vi "PrefValToXMLArray.vi"(8 "error in (no error)":errorcluster, 11 "Preferences in":refnum<class "SetListPrefs.lvclass">) -> (0 "error out":errorcluster, 2 "PrefXML":string[](array[string]), 3 "Preferences out":refnum<class "SetListPrefs.lvclass">)   [LabVIEW 2013, in "SetListPrefs.lvclass"]
uses:
  SetListPrefs.lvclass
  PrefCluster.ctl
  <vilib>/Utility/miscctls.llb/LVRectTypeDef.ctl
  SetListPrefs.lvclass/SetListPrefs.ctl
panel:
  out "PrefCluster":T1
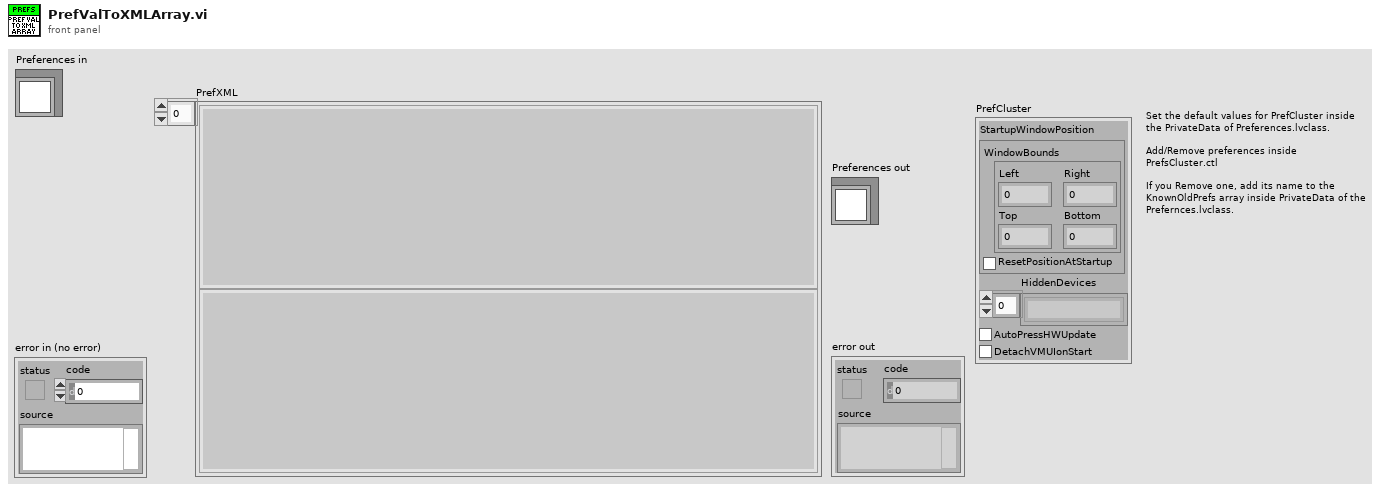
[diagram p1: front panel]
types:
  T1 = typedef "SetListPrefs.lvclass/PrefCluster.ctl" = cluster{"StartupWindowPosition":cluster{"WindowBounds":T2, "ResetPositionAtStartup":bool}, "HiddenDevices":string[], "AutoPressHWUpdate":bool, "DetachVMUIonStart":bool}
  T2 = typedef "LVRectTypeDef.ctl" = cluster{"Left":i16, "Top":i16, "Right":i16, "Bottom":i16}
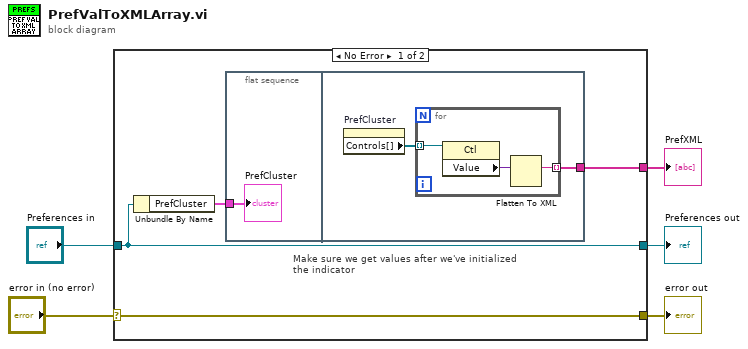
[diagram p0: block diagram]
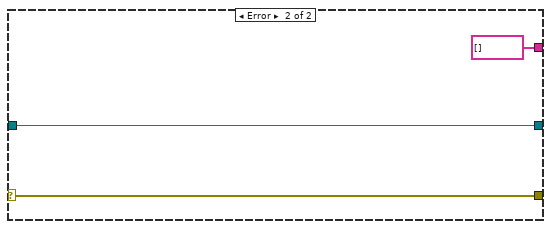
[diagram p2: hidden frame]
diagram:
  n1 = case shown="No Error" "error in (no error)" {
    selector: "error in (no error)" -> [w9 w18]
    tunnel: [w9 w18] -> w4
    tunnel: [w8 w17] -> w2
    tunnel: "Preferences in" -> [w8 w17]
    tunnel: [w6 string[] []] -> w1
    frame No Error {
      n2 = Unbundle By Name(w8) -> ("PrefCluster"=w7:T1)
      n3 = flat-sequence "Make sure we get values after we've initialized the indicator" {
        tunnel: w7 -> [w10]
        tunnel: [w11] -> w6
        frame #0 {
          "PrefCluster" <- w10
        }
        frame #1 {
          n4 = property on="PrefCluster" class="Clust (strict)"() -> ("Controls[]"=w12:refnum<vi>[])  [unwired: 2 in, 2 out]
          n5 = for {
            tunnel: w12 -> [w15] mode=indexing
            tunnel: [w13] -> w11 mode=indexing
            n6 = property class="Ctl"(reference=w15) -> ("Value"=w14:variant)  [unwired: 1 in, 2 out]
            n7 = Flatten To XML(anything=w14) -> (xml string=w13:string)
          }
        }
      }
    }
    frame Error {
    }
  }
  "error out" <- w4
  "Preferences out" <- w2
  "PrefXML" <- w1
